vi "Point To Row Column.vi"(8 "error in (no error)":errorcluster, 10 "Point":T1, 11 "TreeControl in":refnum<class "TreeControl.lvclass">) -> (0 "error out":errorcluster, 1 "Tag":string, 2 "In Bounds?":bool, 3 "TreeControl out":refnum<class "TreeControl.lvclass">, 4 "Column":i32, 5 "In Symbol?":bool)   [LabVIEW 2015, in "TreeControl.lvclass"]
doc: "Converts a pixel coordinate to a tag-column pair in the coordinates of the control. This method also returns whether the point is inside the bounds of the content rectangle and whether the point is within the custom symbol of the cell. The method returns the tag TREE_COLUMN_HEADERS when you wire a point that is within the tree's column headers.\n\n <b>Note</b> The <b>Point to Row Column</b> method does not return an error for points that lie within a control but outside of the actual cell area for that control, such as the scroll bar. Use the <b>InBounds</b> parameter to verify that a point lies within the cell area of a control.\n\nQControl Class wrapper around the <b>TreeControl : Point to Row Column Method</b>.\n<b> </b> <b> </b>\n©2016 Q Software Innovations, LLC (QSI)\nwritten by Quentin Alldredge\nproduced in LabVIEW 2015\n\nsupport@qsoftwareinnovations.com\nwww.qsoftwareinnovations.com\n\nAll rights reserved.\n\nRedistribution and use in source and binary forms, with or without modification, are permitted provided that the following conditions are met:\n\n * Redistributions of source code must retain the above copyright notice, this list of conditions and the following disclaimer.\n * Redistributions in binary form must reproduce the above copyright notice, this list of conditions and the following disclaimer in the documentation and/or other materials provided with the distribution.\n * Neither the name of Q Software Innovations, LLC. nor the names of its contributors may be used to endorse or promote products derived from this software without specific prior written permission.\n\nTHIS SOFTWARE IS PROVIDED BY THE COPYRIGHT HOLDERS AND CONTRIBUTORS \"AS IS\" AND ANY EXPRESS OR IMPLIED WARRANTIES, INCLUDING, BUT NOT LIMITED TO, THE IMPLIED WARRANTIES OF MERCHANTABILITY AND FITNESS FOR A PARTICULAR PURPOSE ARE DISCLAIMED. IN NO EVENT SHALL THE COPYRIGHT OWNER OR CONTRIBUTORS BE LIABLE FOR ANY DIRECT, INDIRECT, INCIDENTAL, SPECIAL, EXEMPLARY, OR CONSEQUENTIAL DAMAGES (INCLUDING, BUT NOT LIMITED TO, PROCUREMENT OF SUBSTITUTE GOODS OR SERVICES; LOSS OF USE, DATA, OR PROFITS; OR BUSINESS INTERRUPTION) HOWEVER CAUSED AND ON ANY THEORY OF LIABILITY, WHETHER IN CONTRACT, STRICT LIABILITY, OR TORT (INCLUDING NEGLIGENCE OR OTHERWISE) ARISING IN ANY WAY OUT OF THE USE OF THIS SOFTWARE, EVEN IF ADVISED OF THE POSSIBILITY OF SUCH DAMAGE."
uses:
  TreeControl.lvclass
  <vilib>/Utility/miscctls.llb/LVPositionTypeDef.ctl
  TreeControl.lvclass/TreeControl.ctl
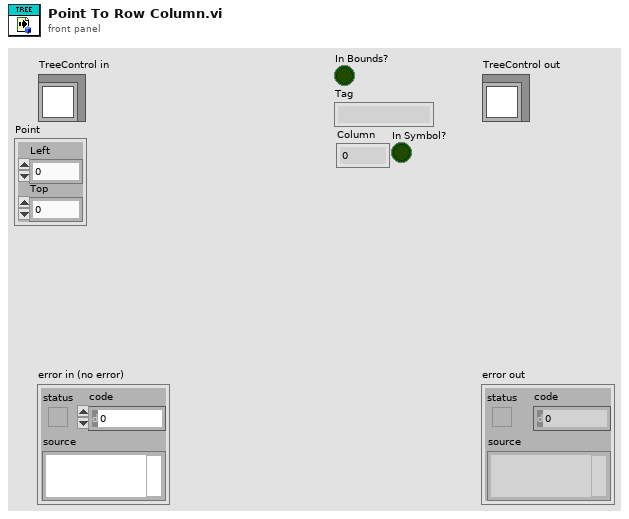
[diagram p1: front panel]
types:
  T1 = typedef "LVPositionTypeDef.ctl" = cluster{"Left":i32, "Top":i32}
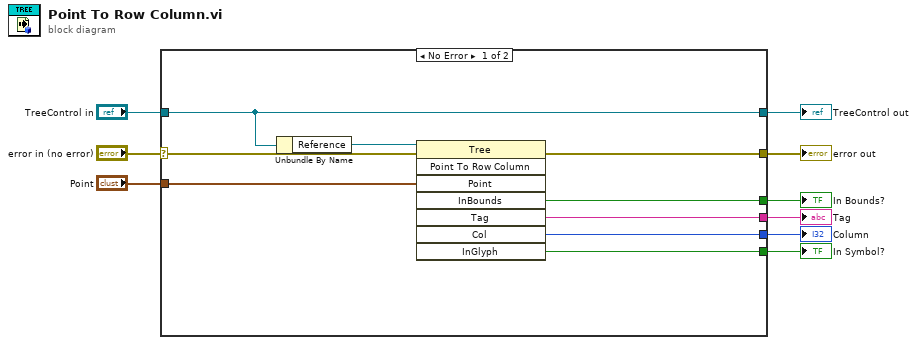
[diagram p0: block diagram]
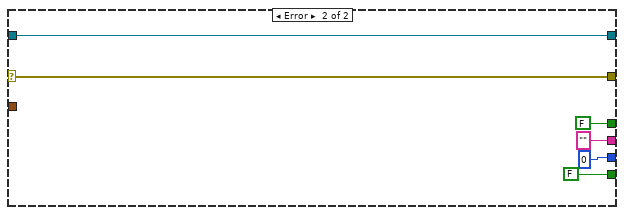
[diagram p2: hidden frame]
diagram:
  n1 = case shown="No Error" "error in (no error)" {
    selector: "error in (no error)" -> [w18 w24]
    tunnel: [w17 w24] -> w8
    tunnel: [w16 w23] -> w6
    tunnel: "TreeControl in" -> [w16 w23]
    tunnel: "Point" -> [w14 _]
    tunnel: [w13 FALSE ("InBounds")] -> w4
    tunnel: [w12 "" ("Tag")] -> w3
    tunnel: [w11 0 ("Col")] -> w2
    tunnel: [w10 FALSE ("InGlyph")] -> w1
    frame No Error {
      n2 = Unbundle By Name(w16) -> ("Reference"=w15:refnum<vi>)
      n3 = invoke class="Tree" method="Point To Row Column"(reference=w15, error in=w18, "Point"=w14) -> (error out=w17:errorcluster, "InBounds"=w13:bool, "Tag"=w12:string, "Col"=w11:i32, "InGlyph"=w10:bool)  [unwired: 5 in, 3 out]
    }
    frame Error {
    }
  }
  "error out" <- w8
  "TreeControl out" <- w6
  "In Bounds?" <- w4
  "Tag" <- w3
  "Column" <- w2
  "In Symbol?" <- w1
